vi "encodeFloat64.vi"(3 "Float64":dbl) -> (1 "MessagePack":u8[](array[numeric]) format="%.0x")   [LabVIEW 2015, in "MsgPack.lvlib"]
uses:
  MsgPack.lvlib
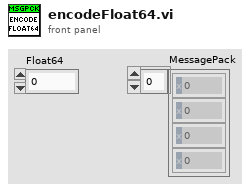
[diagram p1: front panel]
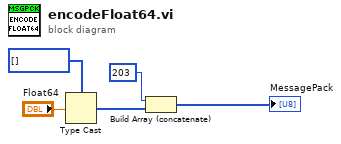
[diagram p0: block diagram]
diagram:
  n1 = Type Cast(type=u8[] [], x="Float64") -> (*(type *) &x=w2:u8[])
  n2 = Build Array (concatenate)(u8 203, w2) -> (→"MessagePack":u8[])
